vi "Note.vi"(1 "通知器 2":refnum<notifier>) -> (0 "布尔":bool)   [LabVIEW 2019]
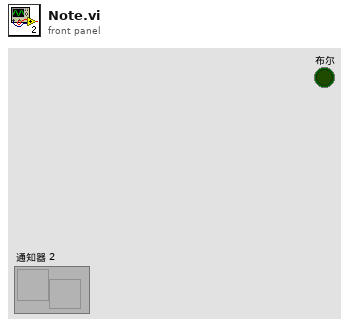
[diagram p1: front panel]
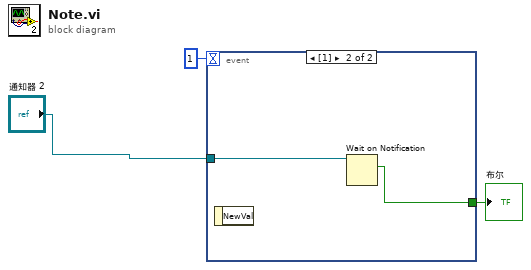
[diagram p0: block diagram]
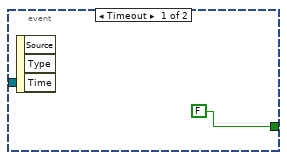
[diagram p2: hidden frame]
diagram:
  n1 = event shown="[1]" {
    selector: _ -> [_ _]
    dyn-events: _ -> [_ _]
    timeout: 1 -> [_ _]
    tunnel: "通知器 2" -> [_ w6]
    tunnel: [FALSE w5] -> w2
    event Timeout {
      n2 = event-data() -> ()  [unwired: 1 in, 3 out]
    }
    event #1 (no event record) {
      n3 = event-data() -> ()  [unwired: 1 in, 1 out]
      n4 = Wait on Notification(notifier=w6) -> (notification=w5:bool)  [unwired: 3 in, 3 out]
    }
  }
  "布尔" <- w2
